vi "Actor Core.vi"(8 "error in":errorcluster, 11 "NI Vision Camera in":refnum<class "NI Vision Camera.lvclass">) -> (0 "error out":errorcluster, 3 "Actor out":refnum<class "Actor.lvclass">)   [LabVIEW 2014, in "NI Vision Camera.lvclass"]
doc: "(<B>Filename</B>: Actor Framework.lvlib:Actor.lvclass:Actor Core.vi)\n\nReceives messages to the actor, reacts to them, and initiates any error handling that may shut the actor down.\n\nDescendant classes may override this VI to append parallel tasks for the actor to complete while it handles messages. Overrides use the Call Parent Method node."
uses:
  NI Vision Camera.lvclass
  <vilib>/ActorFramework/Actor/Actor.lvclass
  <vilib>/ActorFramework/Actor/Actor.lvclass/Actor.ctl
  <vilib>/ActorFramework/Message Enqueuer/Message Enqueuer.lvclass/Message Enqueuer.ctl
  Framework/Interfaces/Pipelined Actor/Pipelined Actor Messages/Do Main Action Msg/Do Main Action Msg.lvclass/Do Main Action Msg.ctl
  NI Vision Camera Device/Configuration.ctl
  NI Vision Camera Messages/Set Camera Configuration Msg/Set Camera Configuration Msg.lvclass/Set Camera Configuration Msg.ctl
  Framework/Model/Data/Data2D/Data2D.lvclass
  <vilib>/ActorFramework/Message Enqueuer/Init from Existing Queue.vi
  <vilib>/ActorFramework/Message Enqueuer/Enqueue.vi
  <vilib>/ActorFramework/Message Priority Queue/Priority Enqueue.vi
  <vilib>/ActorFramework/Message Enqueuer/Message Enqueuer.lvclass
  Framework/Model/Data/AbstractData/AbstractData.lvclass
  Framework/Interfaces/Pipelined Actor/Pipelined Actor Messages/Do Main Action Msg/Do Main Action Msg.lvclass
  NI Vision Camera Messages/Set Camera Configuration Msg/Set Camera Configuration Msg.lvclass
  Framework/Hardware/ReadoutDevice/ReadoutDevice.lvclass
  Framework/Interfaces/Viewable Actor/Viewable Actor.lvclass
  Framework/Interfaces/Observable Actor/Observable Actor.lvclass
  NI Vision Camera Device/NI Vision Camera Device.lvclass
panel:
  in  "Gain (dB)":dbl min=0.0 max=20.0
  in  "Exposure (us)":dbl=20.0 min=20.0 max=1000000.0
  out "Stop":bool=TRUE
  out "Preview":dbl[][](graph)
  out "isShow":bool=TRUE
  in  "Read":bool
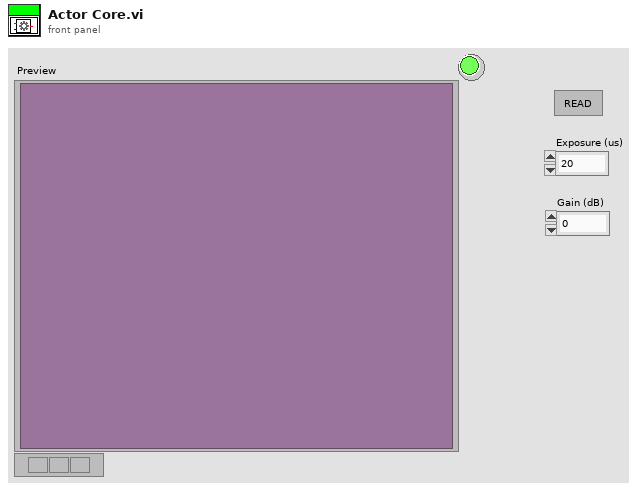
[diagram p1: front panel]
types:
  T1 = typedef "Observable Actor.lvlib/Observable Actor.lvclass/Observer.ctl" = refnum<queue>
  T2 = typedef "NI Vision Camera Device.lvclass/Configuration.ctl" = cluster{"Exposure":dbl, "Gain":dbl}
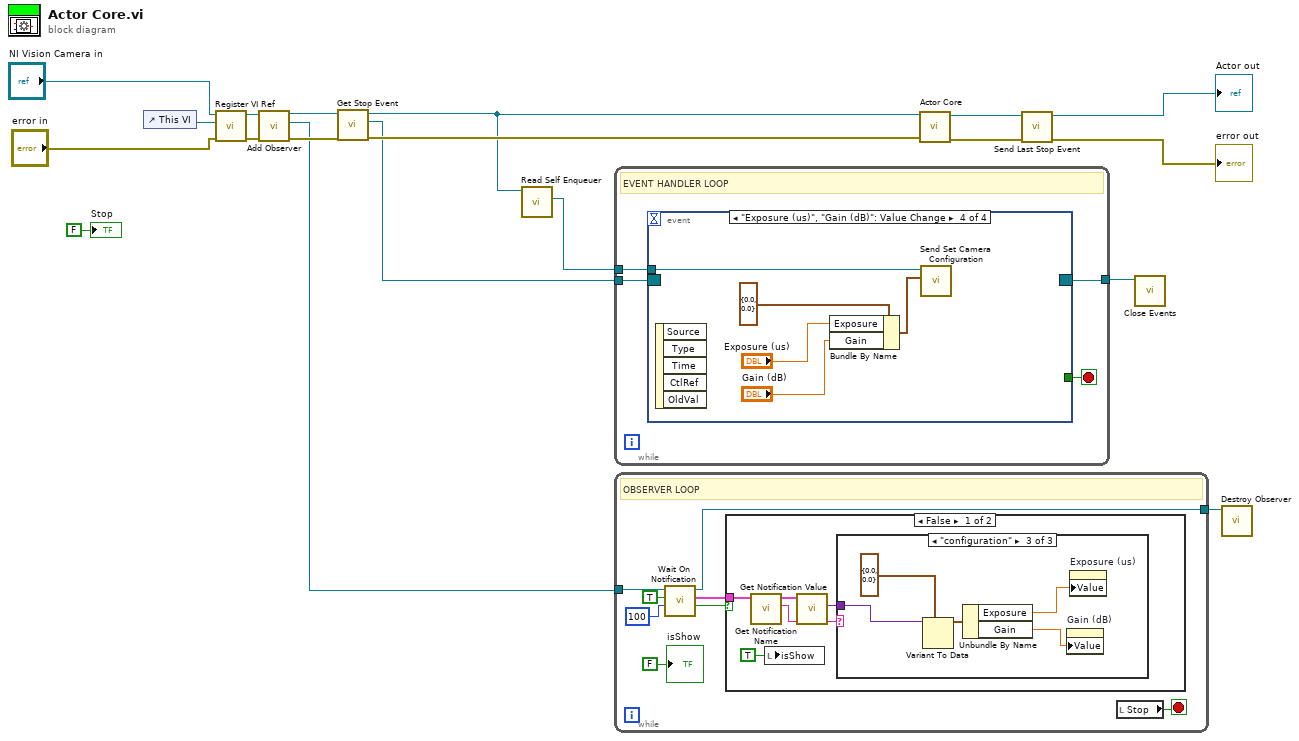
[diagram p0: block diagram]
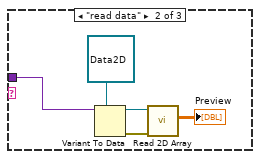
[diagram p3: hidden frame]
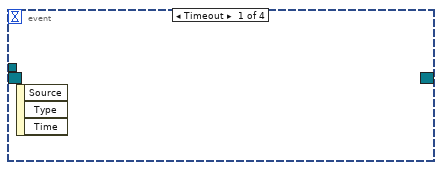
[diagram p5: hidden frame]
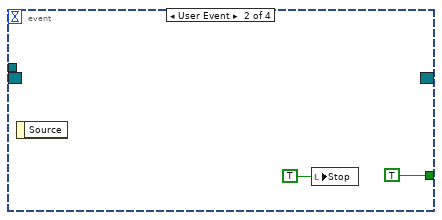
[diagram p6: hidden frame]
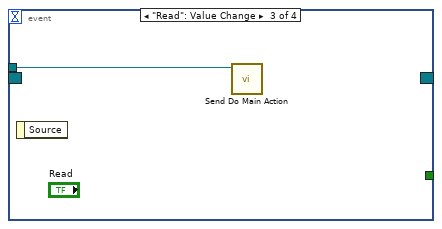
[diagram p7: hidden frame]
diagram:
  n1 = control-ref of="This VI"() -> (w18:refnum<vi>)
  n2 = call "Register VI Ref.vi"("error in (no error)"="error in", "VI ref"=w18, "Viewable Actor in"="NI Vision Camera in") -> ("error out"=w15:errorcluster, "Viewable Actor out"=w16:refnum<class "NI Vision Camera.lvclass">)  [unwired: 7 in]
  n3 = call-dynamic "Add Observer.vi"("error in (no error)"=w15, "Observable Actor in"=w16) -> ("error out"=w19:errorcluster, "new observer"=w14:T1, "Observable Actor out"=w13:refnum<class "NI Vision Camera.lvclass">)  [unwired: 7 in]
  n4 = call-dynamic "Get Stop Event.vi"("error in (no error)"=w19, "Observable Actor in"=w13) -> ("error out"=w12:errorcluster, "Events"=w11:refnum<event-registration>, "Observable Actor out"=w5:refnum<class "NI Vision Camera.lvclass">)  [unwired: 7 in]
  n5 = call <vilib>:"Read Self Enqueuer.vi"("Actor"=w5) -> ("Self Enqueuer"=w17:refnum<class "Message Enqueuer.lvclass">)  [unwired: 10 in]
  n6 = while {
    tunnel: w11 -> [w23]
    tunnel: w17 -> [w22]
    tunnel: [w21] -> w10
    stop <- w20 stop-if-true
    # "EVENT HANDLER LOOP"
    n7 = event shown="[3] \"Exposure (us)\", \"Gain (dB)\": Value Change" {
      selector: w23 -> [_ _ _ _]
      dyn-events: [_ _ _ _] -> w21
      timeout: _ -> [_ _ _ _]
      tunnel: w22 -> [_ _ w26 w31]
      tunnel: [_ TRUE _ _] -> w20
      event Timeout {
        n8 = event-data() -> ()  [unwired: 1 in, 3 out]
      }
      event User Event {
        n9 = event-data() -> ()  [unwired: 1 in, 1 out]
        n10 = local write "Stop"(TRUE ("Stop")) -> ()
      }
      event "Read": Value Change {
        n11 = event-data() -> ()  [unwired: 1 in, 1 out]
        n12 = call "Send Do Main Action.vi"("Message Enqueuer"=w26) -> ()  [unwired: 9 in, 2 out]
      }
      event "Exposure (us)", "Gain (dB)": Value Change {
        n13 = event-data() -> ()  [unwired: 1 in, 5 out]
        n14 = Bundle By Name(cluster=T2 {"Exposure"=0.0, "Gain"=0.0} ("Configuration"), "Exposure"="Exposure (us)", "Gain"="Gain (dB)") -> (w28:T2)
        n15 = call "Send Set Camera Configuration.vi"("Configuration"=w28, "Message Enqueuer"=w31) -> ()  [unwired: 8 in, 2 out]
      }
    }
  }
  n16 = while {
    tunnel: w14 -> [w34]
    tunnel: [w33] -> w7
    stop <- w39 stop-if-true
    # "OBSERVER LOOP"
    n17 = call "Wait On Notification.vi"("timeout in ms (-1)"=100, "ignore previous (F)"=TRUE, "observer in"=w34) -> ("timed out?"=w35:bool, "notification"=w36:cluster{"value":variant, "name":string}, "observer out"=w33:T1)  [unwired: 5 in, 1 out]
    n18 = case shown="False" w35 {
      tunnel: w36 -> [w43 _]
      frame False {
        n19 = call "Get Notification Name.vi"("notification in"=w43) -> ("name"=w41:string, "notification out"=w42:cluster{"value":variant, "name":string})  [unwired: 9 in]
        n20 = local write "isShow"(TRUE ("isShow")) -> ()
        n21 = call "Get Notification Value.vi"("notification in"=w42) -> ("data"=w44:variant)  [unwired: 7 in, 1 out]
        n22 = case shown="\"configuration\"" w41 {
          tunnel: w44 -> [_ w49 w54]
          frame "False", Default {
          }
          frame "read data" {
            n23 = Variant To Data(type=refnum<class "Data2D.lvclass"> refnum ("Data2D.lvclass"), Variant=w49) -> (data=w47:refnum<class "Data2D.lvclass">, error out=w46:errorcluster)  [unwired: 1 in]
            n24 = call "Read 2D Array.vi"("error in (no error)"=w46, "Data2D in"=w47) -> ("2D Array"=→"Preview":dbl[][])  [unwired: 7 in, 2 out]
          }
          frame "configuration" {
            n25 = Variant To Data(type=T2 {"Exposure"=0.0, "Gain"=0.0} ("Configuration"), Variant=w54) -> (data=w53:T2)  [unwired: 1 in, 1 out]
            n26 = Unbundle By Name(w53) -> ("Exposure"=w52:dbl, "Gain"=w51:dbl)
            n27 = property on="Gain (dB)" class="DigNum (strict)"("Value"=w51) -> ()  [unwired: 2 in, 2 out]
            n28 = property on="Exposure (us)" class="DigNum (strict)"("Value"=w52) -> ()  [unwired: 2 in, 2 out]
          }
        }
      }
      frame True {
      }
    }
    n29 = local read "Stop"() -> (w39:bool)
    "isShow" <- FALSE ("Boolean")
  }
  n30 = call-parent "Actor Core.vi"("error in"=w12, "Actor in"=w5) -> ("error out"=w8:errorcluster, "Actor out"=w9:refnum<class "Actor.lvclass">)  [unwired: 8 in]
  n31 = call "Send Last Stop Event.vi"("error in (no error)"=w8, "Actor in"=w9) -> ("error out"=→"error out":errorcluster, "Actor  out"=→"Actor out":refnum<class "Actor.lvclass">)  [unwired: 8 in]
  n32 = call "Close Events.vi"("events"=w10) -> ()  [unwired: 11 in]
  n33 = call "Destroy Observer.vi"("observer in"=w7) -> ()  [unwired: 11 in]
  "Stop" <- FALSE ("Stop")
